vi "_TestOFFRegion.vi"(0 "VISA Resource Name":refnum<visa-resource-name>, 1 "Project #":string, 2 "Request #":string, 3 "TEST #":string, 4 "ICE":dbl, 5 "VGE":dbl, 6 "VCE":dbl, 7 "error in (no error)":errorcluster) -> (8 "Tdoff (ns)":dbl, 9 "Di (A)":dbl, 10 "Tf (ns)":dbl, 11 "Dt (ns)":dbl, 12 "Di/Dt (A/us)":dbl, 14 "Dv/Dt (V/us)":dbl, 16 "Eoff (uj)":dbl, 17 "Dv (V)":dbl, 19 "Dt (ns) 2":dbl, 20 "DONE Tdoff":bool, 21 "DONE Tf":bool, 22 "DONE Di/Dt OFF":bool, 23 "DONE Dv/Dt OFF":bool, 24 "DONE Eoff":bool, 26 "Waveform Graph":waveform(dbl)[](graph), 27 "error out":errorcluster)   [LabVIEW 2020]
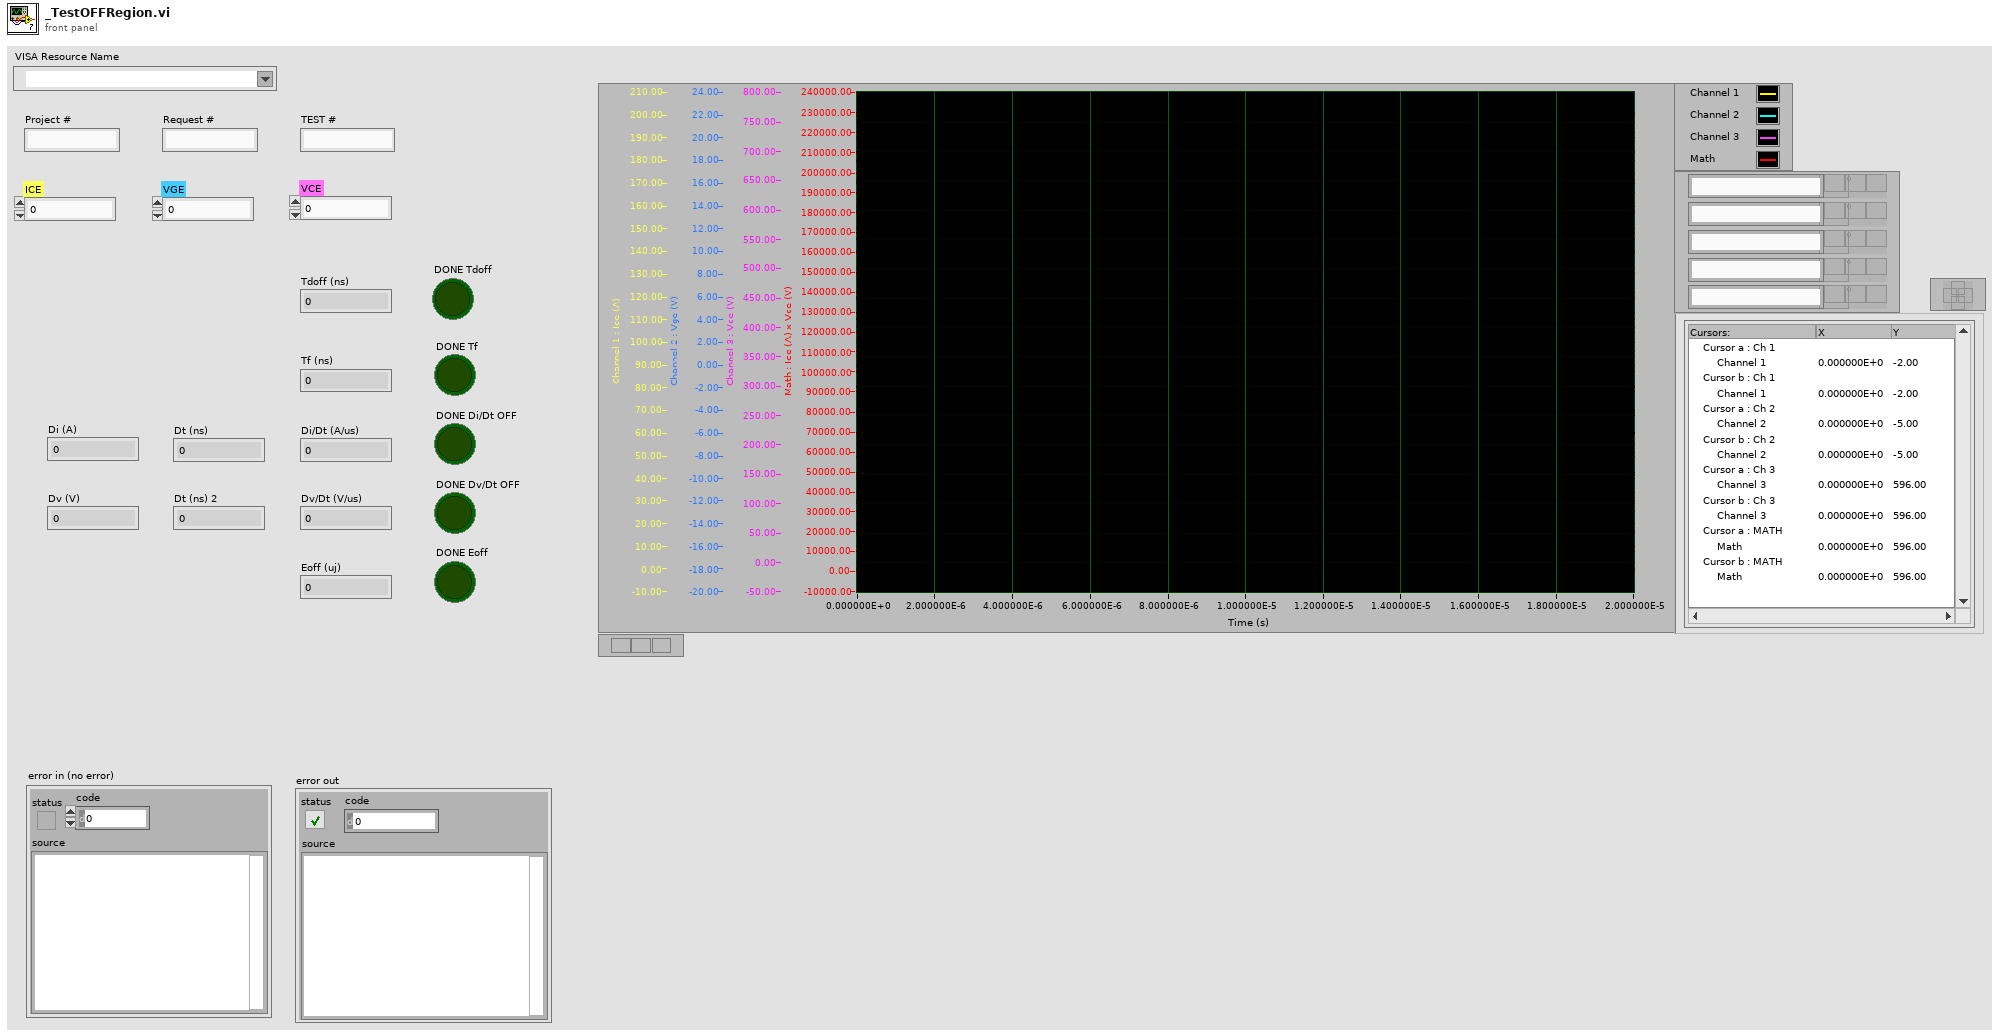
[diagram p1: front panel]
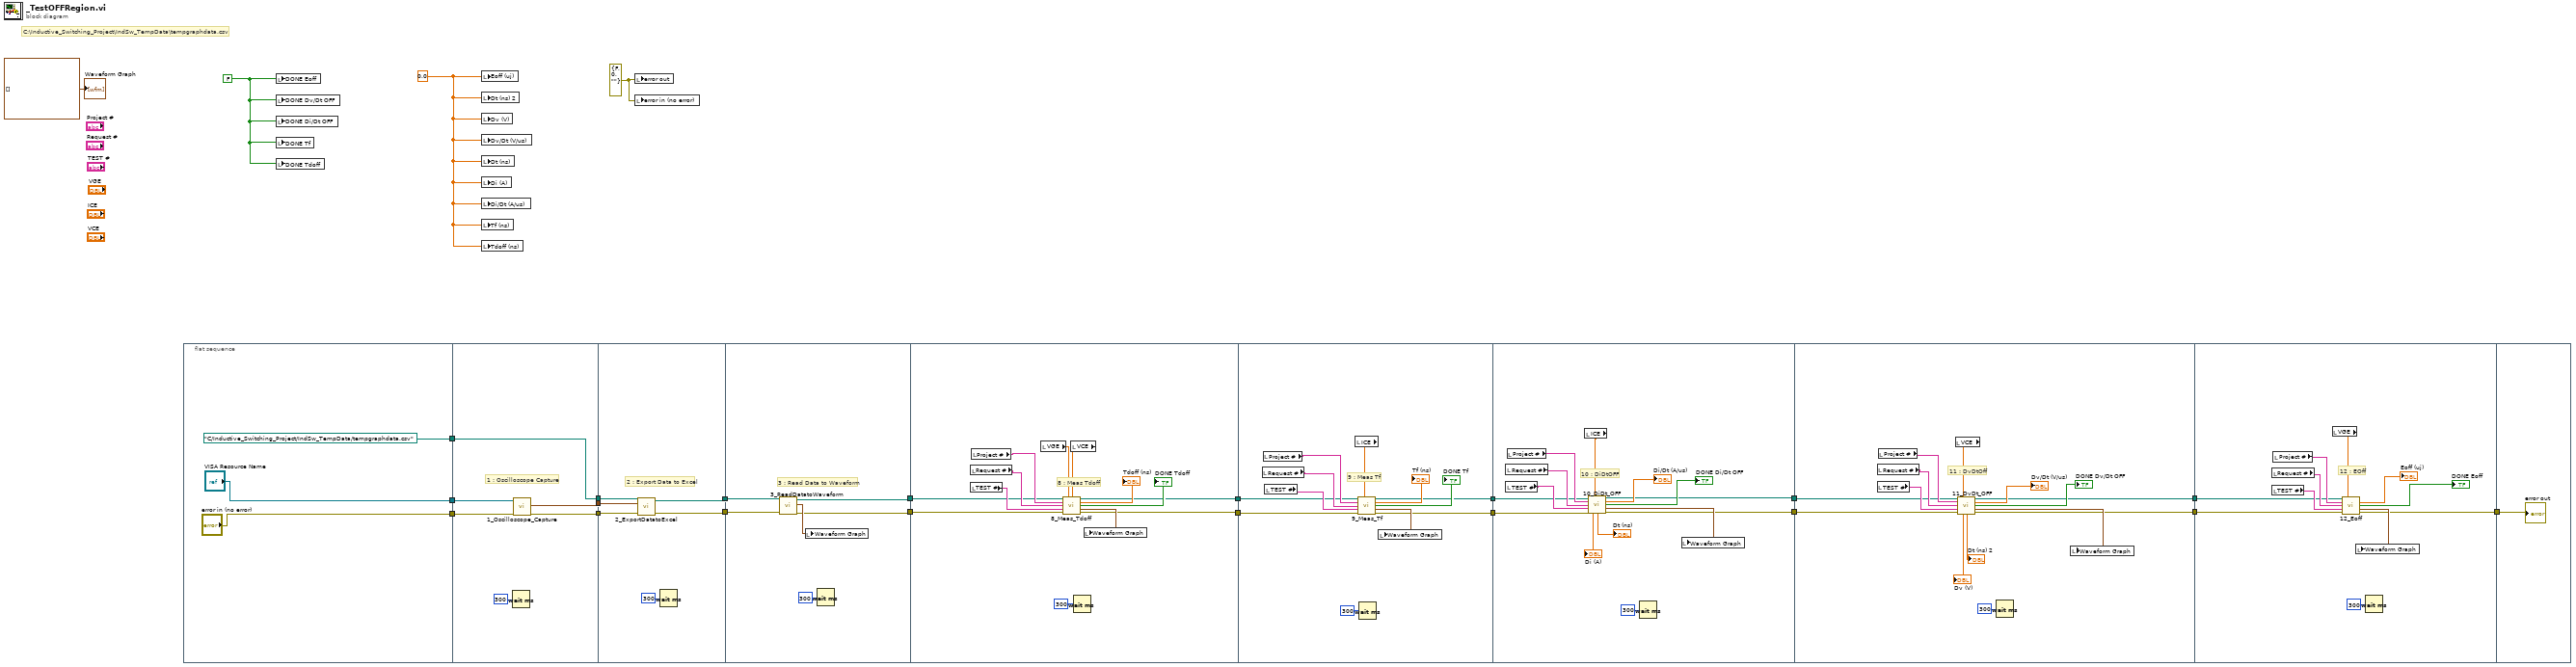
[diagram p0: block diagram]
diagram:
  w20 = errorcluster {"status"=FALSE, "code"=0, "source"=""} ("error out")
  w21 = 0.0 ("Eoff (uj)")
  w22 = FALSE ("DONE Eoff")
  # "C:\\Inductive_Switching_Project\\IndSw_TempData\\tempgraphdata.csv"
  n1 = flat-sequence {
    tunnel: [path "C:/Inductive_Switching_Project/IndSw_TempData/tempgraphdata.csv" ("file path (IN)")] -> w3
    tunnel: ["error in (no error)"] -> w2
    tunnel: ["VISA Resource Name"] -> w1
    tunnel: [w28] -> w6
    tunnel: [w27] -> w5
    tunnel: [w32] -> w4
    tunnel: w3 -> [w32]
    tunnel: w2 -> [w30]
    tunnel: w1 -> [w29]
    tunnel: [w34] -> w8
    tunnel: [w33] -> w7
    tunnel: w6 -> [w37]
    tunnel: w5 -> [w36]
    tunnel: w4 -> [w35]
    tunnel: [w39] -> w10
    tunnel: [w40] -> w9
    tunnel: w8 -> [w42]
    tunnel: w7 -> [w41]
    tunnel: [w46] -> w12
    tunnel: [w45] -> w11
    tunnel: w10 -> [w48]
    tunnel: w9 -> [w47]
    tunnel: [w59] -> w14
    tunnel: [w58] -> w13
    tunnel: w12 -> [w61]
    tunnel: w11 -> [w60]
    tunnel: [w71] -> w16
    tunnel: [w70] -> w15
    tunnel: w14 -> [w73]
    tunnel: w13 -> [w72]
    tunnel: [w85] -> w18
    tunnel: [w84] -> w17
    tunnel: w16 -> [w87]
    tunnel: w15 -> [w86]
    tunnel: [w98] -> w19
    tunnel: w18 -> [w100]
    tunnel: w17 -> [w99]
    tunnel: w19 -> [w109]
    frame #0 {
    }
    frame #1 {
      # "1 : Oscilloscope Capture"
      n2 = Wait (ms)(milliseconds to wait=u32 300) -> ()  [unwired: 1 out]
      n3 = call "1_Oscilloscope_Capture.vi"("error in (no error)"=w30, "VISA Resource Name"=w29) -> ("error out"=w28:errorcluster, "Waveform Graph"=w27:waveform(dbl)[])  [unwired: 7 in, 1 out]
    }
    frame #2 {
      # "2 : Export Data to Excel"
      n4 = call "2_ExportDatatoExcel.vi"("error in (no error)"=w37, "Waveform Graph"=w36, "file path (IN)"=w35) -> ("error out"=w34:errorcluster, "file path (OUT)"=w33:path)  [unwired: 7 in]
      n5 = Wait (ms)(milliseconds to wait=u32 300) -> ()  [unwired: 1 out]
    }
    frame #3 {
      # "3 : Read Data to Waveform"
      n6 = call "3_ReadDatatoWaveform.vi"("error in (no error)"=w42, "file path (IN)"=w41) -> ("error out"=w40:errorcluster, "Waveform Graph"=w44:waveform(dbl)[], "file path (OUT)"=w39:path)  [unwired: 3 in, 4 out]
      n7 = local write "Waveform Graph"(w44) -> ()
      n8 = Wait (ms)(milliseconds to wait=u32 300) -> ()  [unwired: 1 out]
    }
    frame #4 {
      # "8 : Meas Tdoff"
      n9 = local read "Request #"() -> (w52:string)
      n10 = local read "TEST #"() -> (w53:string)
      n11 = local read "Project #"() -> (w51:string)
      n12 = local read "VGE"() -> (w54:dbl)
      n13 = local read "VCE"() -> (w55:dbl)
      n14 = call "8_Meas_Tdoff.vi"("file path (IN)"=w48, "VGE"=w54, "VCE"=w55, "Project #"=w51, "Request #"=w52, "TEST #"=w53, "error in (no error)"=w47) -> ("file path (OUT)"=w46:path, "Tdoff (ns)"=→"Tdoff (ns)":dbl, "DONE Tdoff"=→"DONE Tdoff":bool, "OFF Region"=w50:waveform(dbl)[], "error out"=w45:errorcluster)  [unwired: 4 in]
      n15 = Wait (ms)(milliseconds to wait=u32 300) -> ()  [unwired: 1 out]
      n16 = local write "Waveform Graph"(w50) -> ()
    }
    frame #5 {
      # "9 : Meas Tf"
      n17 = local read "Request #"() -> (w65:string)
      n18 = local read "Project #"() -> (w64:string)
      n19 = local read "TEST #"() -> (w66:string)
      n20 = local read "ICE"() -> (w69:dbl)
      n21 = call "9_Meas_Tf.vi"("file path (IN)"=w61, "ICE"=w69, "Project #"=w64, "Request #"=w65, "TEST #"=w66, "error in (no error)"=w60) -> ("file path (OUT)"=w59:path, "Tf (ns)"=→"Tf (ns)":dbl, "DONE Tf"=→"DONE Tf":bool, "OFF Region"=w63:waveform(dbl)[], "error out"=w58:errorcluster)  [unwired: 5 in]
      n22 = Wait (ms)(milliseconds to wait=u32 300) -> ()  [unwired: 1 out]
      n23 = local write "Waveform Graph"(w63) -> ()
    }
    frame #6 {
      # "10 : DiDtOFF"
      n24 = local read "Request #"() -> (w77:string)
      n25 = local read "TEST #"() -> (w78:string)
      n26 = local read "Project #"() -> (w76:string)
      n27 = local read "ICE"() -> (w79:dbl)
      n28 = call "10_DiDt_OFF.vi"("file path (IN)"=w73, "ICE"=w79, "Project #"=w76, "Request #"=w77, "TEST #"=w78, "error in (no error)"=w72) -> ("file path (OUT)"=w71:path, "Di/Dt (A/us)"=→"Di/Dt (A/us)":dbl, "DONE Di/Dt OFF"=→"DONE Di/Dt OFF":bool, "OFF Region"=w75:waveform(dbl)[], "Di (A)"=→"Di (A)":dbl, "Dt (ns)"=→"Dt (ns)":dbl, "error out"=w70:errorcluster)  [unwired: 3 in]
      n29 = Wait (ms)(milliseconds to wait=u32 300) -> ()  [unwired: 1 out]
      n30 = local write "Waveform Graph"(w75) -> ()
    }
    frame #7 {
      # "11 : DvDtOff"
      n31 = local read "Request #"() -> (w91:string)
      n32 = local read "TEST #"() -> (w92:string)
      n33 = local read "Project #"() -> (w90:string)
      n34 = local read "VCE"() -> (w93:dbl)
      n35 = call "11_DvDt_OFF.vi"("file path (IN)"=w87, "VCE"=w93, "Project #"=w90, "Request #"=w91, "TEST #"=w92, "error in (no error)"=w86) -> ("file path (OUT)"=w85:path, "Dv/Dt (V/us)"=→"Dv/Dt (V/us)":dbl, "DONE Dv/Dt OFF"=→"DONE Dv/Dt OFF":bool, "OFF Region"=w89:waveform(dbl)[], "Dv (V)"=→"Dv (V)":dbl, "Dt (ns)"=→"Dt (ns) 2":dbl, "error out"=w84:errorcluster)  [unwired: 3 in]
      n36 = Wait (ms)(milliseconds to wait=u32 300) -> ()  [unwired: 1 out]
      n37 = local write "Waveform Graph"(w89) -> ()
    }
    frame #8 {
      # "12 : EOff"
      n38 = local read "Request #"() -> (w104:string)
      n39 = local read "TEST #"() -> (w105:string)
      n40 = local read "Project #"() -> (w103:string)
      n41 = local read "VGE"() -> (w106:dbl)
      n42 = call "12_Eoff.vi"("file path (IN)"=w100, "VGE"=w106, "Project #"=w103, "Request #"=w104, "TEST #"=w105, "error in (no error)"=w99) -> ("Eoff (uj)"=→"Eoff (uj)":dbl, "DONE Eoff"=→"DONE Eoff":bool, "OFF Region"=w102:waveform(dbl)[], "error out"=w98:errorcluster)  [unwired: 5 in, 1 out]
      n43 = local write "Waveform Graph"(w102) -> ()
      n44 = Wait (ms)(milliseconds to wait=u32 300) -> ()  [unwired: 1 out]
    }
    frame #9 {
      "error out" <- w109
    }
  }
  n45 = local write "DONE Eoff"(w22) -> ()
  n46 = local write "DONE Dv/Dt OFF"(w22) -> ()
  n47 = local write "DONE Di/Dt OFF"(w22) -> ()
  n48 = local write "DONE Tf"(w22) -> ()
  n49 = local write "DONE Tdoff"(w22) -> ()
  n50 = local write "Eoff (uj)"(w21) -> ()
  n51 = local write "Dt (ns) 2"(w21) -> ()
  n52 = local write "Dv (V)"(w21) -> ()
  n53 = local write "Dv/Dt (V/us)"(w21) -> ()
  n54 = local write "Dt (ns)"(w21) -> ()
  n55 = local write "Di (A)"(w21) -> ()
  n56 = local write "Di/Dt (A/us)"(w21) -> ()
  n57 = local write "Tf (ns)"(w21) -> ()
  n58 = local write "Tdoff (ns)"(w21) -> ()
  n59 = local write "error out"(w20) -> ()
  n60 = local write "error in (no error)"(w20) -> ()
  "Waveform Graph" <- waveform(dbl)[] [] ("Waveform Graph")
